vi "表格字体上色.vi"(8 "错误输入（无错误）":errorcluster, 9 "列":i32, 10 "颜色输入":u32[](array[colorbox]), 11 "Tbl引用句柄":refnum<vi>) -> (0 "错误输出":errorcluster, 3 "引用输出":refnum<vi>)   [LabVIEW 2014, in "表格.lvlib" / "表格上色.lvlib"]
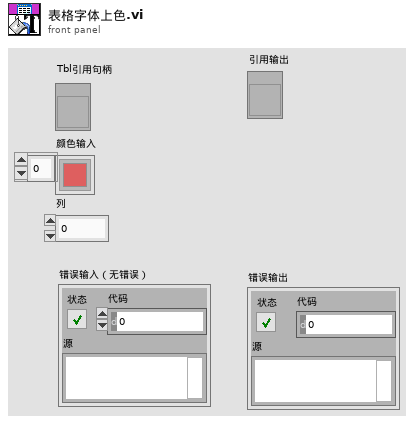
[diagram p1: front panel]
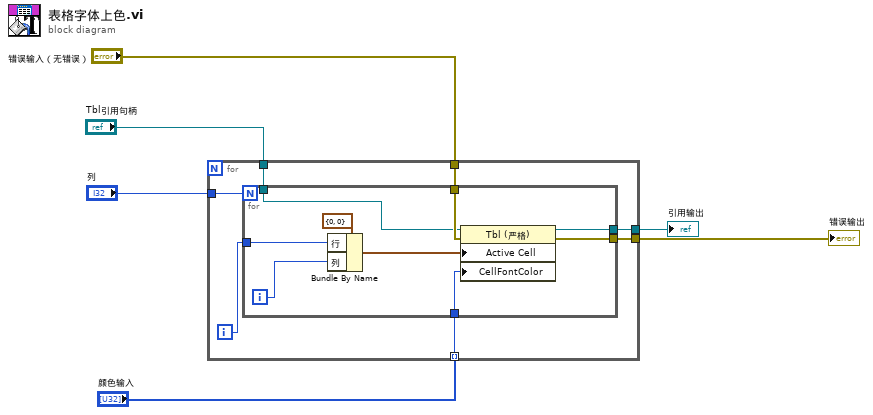
[diagram p0: block diagram]
diagram:
  n1 = for {
    tunnel: "颜色输入" -> [w11] mode=indexing
    tunnel: "列" -> [w13]
    tunnel: "错误输入（无错误）" -> [w10]
    tunnel: [w9] -> w4
    tunnel: [w8] -> w3
    tunnel: "Tbl引用句柄" -> [w7]
    i -> [w12]
    n2 = for {
      N: w13 -> [_]
      tunnel: w12 -> [w21]
      tunnel: w11 -> [w18]
      tunnel: w10 -> [w17]
      tunnel: [w16] -> w9
      tunnel: [w15] -> w8
      tunnel: w7 -> [w14]
      i -> [w20]
      n3 = Bundle By Name(cluster=cluster{"行":i32, "列":i32} {"行"=0, "列"=0}, "行"=w21, "列"=w20) -> (w19:cluster{"行":i32, "列":i32})
      n4 = property class="Tbl (严格)"(reference=w14, error in=w17, "Active Cell"=w19, "CellFontColor"=w18) -> (reference out=w15:refnum<vi>, error out=w16:errorcluster)
    }
  }
  "错误输出" <- w4
  "引用输出" <- w3
